vi "handle_connection.vi"(6 "Log Service":refnum<data-value>, 8 "error in (no error)":errorcluster, 10 "connection":refnum<class "Connection.lvclass">, 11 "Connection Handler in":refnum<class "Connection Handler.lvclass">) -> (0 "error out":errorcluster)   [LabVIEW 2019, in "Socket API.lvlib" / "Connection Handler.lvclass"]
uses:
  Connection Handler.lvclass
  Connection/Connection.lvclass
  Utility API/Log Service/Log Service.lvclass
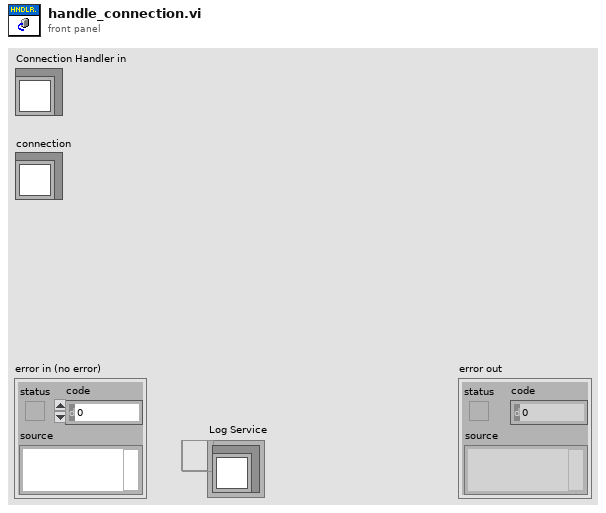
[diagram p1: front panel]
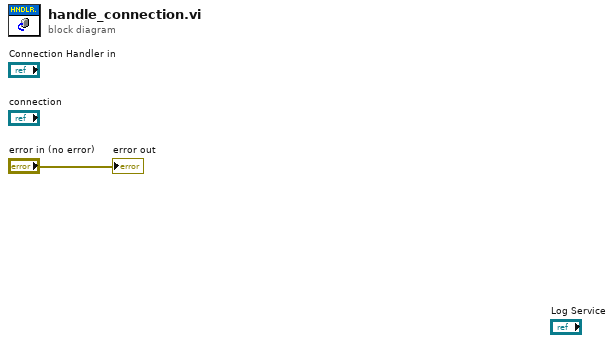
[diagram p0: block diagram]
diagram:
  "error out" <- "error in (no error)"
